vi "Enqueue FGV.vi"(7 "Actions":T1(ring)=enum."Enqueue", 8 "error in":errorcluster, 9 "Message Data":variant, 10 "Message":string, 11 "Priority?":bool) -> (0 "error out":errorcluster, 3 "queue out":refnum<queue>)   [LabVIEW 2020, in "State_Machine_Queue.lvlib"]
doc: "Enqueue single state for the FGV queue based state machine.\n\n\n--------------------\nJuan Navarro\nLab It Studio"
uses:
  State_Machine_Queue.lvlib
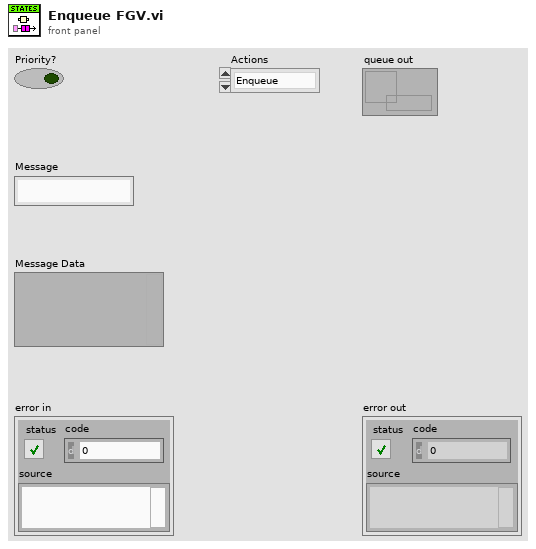
[diagram p1: front panel]
types:
  T1 = enum16{"Obtain", "Enqueue", "Get Queue", "Flush", "Release"}
  T2 = cluster{"Message":string, "Message Data":variant}
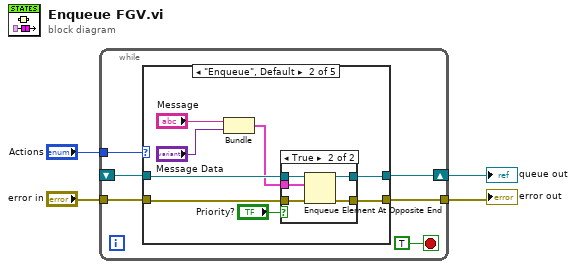
[diagram p0: block diagram]
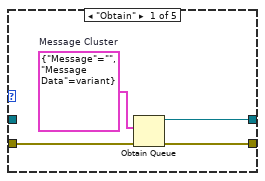
[diagram p2: hidden frame]
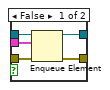
[diagram p3: hidden frame]
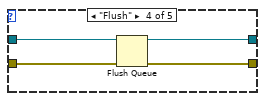
[diagram p5: hidden frame]
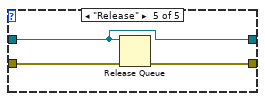
[diagram p6: hidden frame]
diagram:
  n1 = while {
    tunnel: "Actions" -> [w10]
    tunnel: "error in" -> [w9]
    tunnel: [w8] -> w3
    shift-right: [w7] -> w2
    shift-left: _ -> [w6]
    stop <- TRUE stop-if-true
    n2 = case shown="\"Enqueue\", Default" w10 {
      tunnel: w9 -> [w14 w19 w33 w35 w41]
      tunnel: [w13 w21 w33 w37 w40] -> w8
      tunnel: [w12 w22 w34 w38 w39] -> w7
      tunnel: w6 -> [_ w20 w34 w36 w39]
      frame "Obtain" {
        w11 = T2 {"Message"="", "Message Data"=variant}  # Message Cluster
        n3 = Obtain Queue(element data type=w11, error in (no error)=w14) -> (queue out=w12:refnum<queue>, error out=w13:errorcluster)  [unwired: 3 in, 1 out]
      }
      frame "Enqueue", Default {
        n4 = Bundle("Message"="Message", "Message Data"="Message Data") -> (w18:T2)  [unwired: 1 in]
        n5 = case shown="True" "Priority?" {
          tunnel: [w27 w30] -> w22
          tunnel: [w26 w31] -> w21
          tunnel: w20 -> [w25 w29]
          tunnel: w19 -> [w24 w32]
          tunnel: w18 -> [w23 w28]
          frame False {
            n6 = Enqueue Element(queue=w25, element=w23, error in (no error)=w24) -> (queue out=w27:refnum<queue>, error out=w26:errorcluster)  [unwired: 1 in, 1 out]
          }
          frame True {
            n7 = Enqueue Element At Opposite End(queue=w29, element=w28, error in (no error)=w32) -> (queue out=w30:refnum<queue>, error out=w31:errorcluster)  [unwired: 1 in, 1 out]
          }
        }
      }
      frame "Get Queue" {
      }
      frame "Flush" {
        n8 = Flush Queue(queue=w36, error in (no error)=w35) -> (queue out=w38:refnum<queue>, error out=w37:errorcluster)  [unwired: 1 out]
      }
      frame "Release" {
        n9 = Release Queue(queue=w39, error in (no error)=w41) -> (error out=w40:errorcluster)  [unwired: 1 in, 2 out]
      }
    }
  }
  "queue out" <- w2
  "error out" <- w3
